vi "draw circle.vi"(4 "Color":u32(colorbox)=16711680, 6 "error in (no error)":errorcluster, 7 "Drawing Mode (Frame)":u32(ring) items=["Frame", "Fill"], 8 "box size":dbl, 9 "Y":dbl, 10 "X":dbl, 11 "Image In":T1) -> (1 "error out":errorcluster, 3 "Image Out":T1)   [LabVIEW 2019, in "detectedPellet.lvlib"]
uses:
  <vilib>/vision/Image Controls.llb/IMAQ Image.ctl
  detectedPellet.lvlib
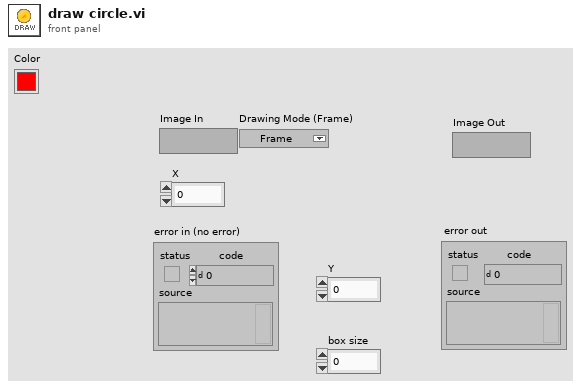
[diagram p1: front panel]
types:
  T1 = typedef "IMAQ Image.ctl" = refnum<image>
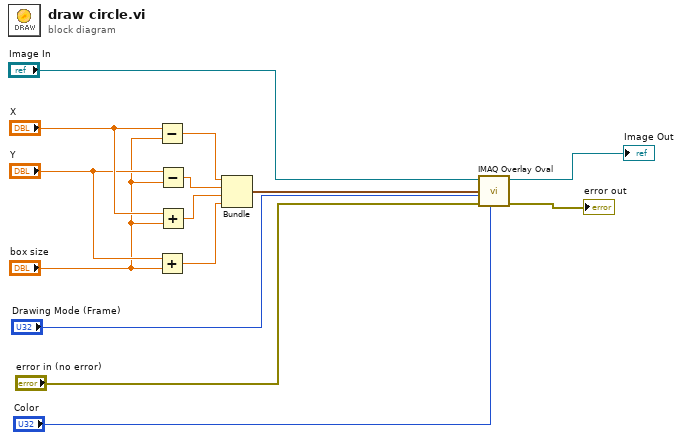
[diagram p0: block diagram]
diagram:
  n1 = Subtract(x="X", y="box size") -> (x-y=w14:dbl)
  n2 = Add(x="Y", y="box size") -> (x+y=w10:dbl)
  n3 = Subtract(x="Y", y="box size") -> (x-y=w12:dbl)
  n4 = Add(x="X", y="box size") -> (x+y=w11:dbl)
  n5 = Bundle(w14, w12, w11, w10) -> (w13:cluster{dbl, dbl, dbl, dbl})  [unwired: 1 in]
  n6 = call "IMAQ Overlay Oval"("Color"="Color", "error in (no error)"="error in (no error)", "Drawing Mode (Frame)"="Drawing Mode (Frame)", "Bounding Rectangle"=w13, "Image"="Image In") -> ("error out"=→"error out":errorcluster, "Image Out"=→"Image Out":T1)  [unwired: 5 in]
